vi "Write COM.vi"(8 "error in (no error)":errorcluster, 10 "COM":refnum<visa-resource-name>, 11 "Osciloscope in":refnum<class "Osciloscope.lvclass">) -> (0 "error out":errorcluster, 3 "Osciloscope out":refnum<class "Osciloscope.lvclass">)   [LabVIEW 2020, in "Osciloscope Tektronix.lvlib" / "Osciloscope.lvclass"]
uses:
  Osciloscope.lvclass
  Osciloscope.lvclass/Osciloscope.ctl
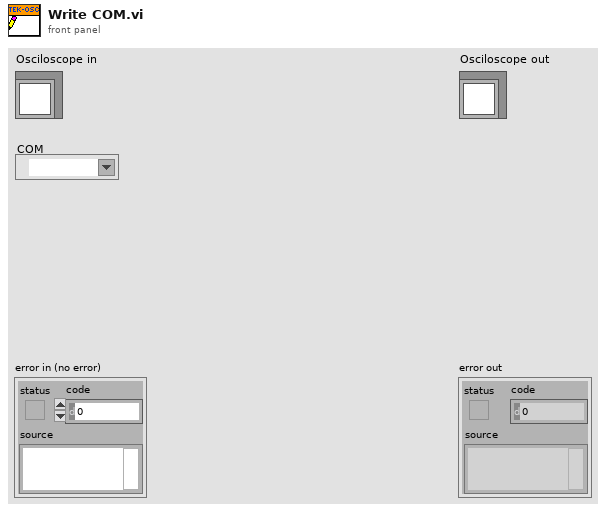
[diagram p1: front panel]
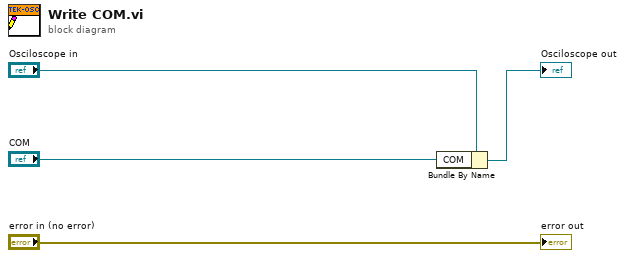
[diagram p0: block diagram]
diagram:
  n1 = Bundle By Name(cluster="Osciloscope in", "COM"="COM") -> (→"Osciloscope out":refnum<class "Osciloscope.lvclass">)
  "error out" <- "error in (no error)"
